vi "FindControl.vi"(5 "Control in":refnum<class "Control.lvclass">, 6 "error in":errorcluster, 9 "Tab in":refnum<class "Tab.lvclass">) -> (0 "error out":errorcluster, 3 "Tab out":refnum<class "Tab.lvclass">, 4 "Tab index":i32)   [LabVIEW 2014, in "Raspberry Pi Compatible Compiler for LabVIEW.lvlib" / "Tab.lvclass"]
uses:
  Tab.lvclass
  Control/Control.lvclass
  PageSelector/PageSelector.lvclass/PageSelector.ctl
  PageSelector/PageSelector.lvclass
  Page/Page.lvclass
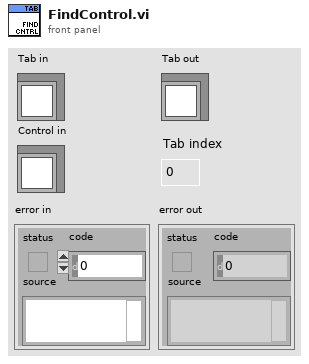
[diagram p1: front panel]
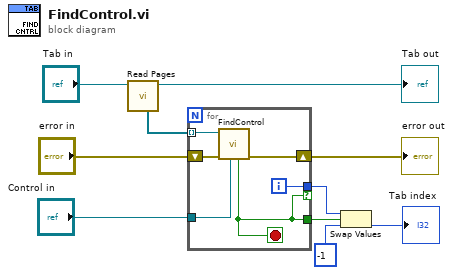
[diagram p0: block diagram]
diagram:
  n1 = call "Read Pages.vi"("PageSelector in"="Tab in") -> ("PageSelector out"=→"Tab out":refnum<class "Tab.lvclass">, "Pages"=w9:refnum<class "Page.lvclass">[])  [unwired: 7 in]
  n2 = for {
    tunnel: w9 -> [w16] mode=indexing
    shift-right: [w14] -> w5
    shift-left: "error in" -> [w15]
    tunnel: "Control in" -> [w13]
    tunnel: [w12] -> w3 if=w11
    tunnel: [w11] -> w4
    i -> [w12]
    stop <- w11 stop-if-true
    n3 = call "FindControl.vi"("Control"=w13, "error in"=w15, "Page in"=w16) -> ("error out"=w14:errorcluster, "On page"=w11:bool)  [unwired: 4 in, 1 out]
  }
  "error out" <- w5
  n4 = Swap Values(12:w3, 13:w4, 14:-1 ("x")) -> (3:→"Tab index":i32)  [unwired: 1 out]
